vi "GetCurrentCharacter.vi"(8 "error in (no error)":errorcluster, 11 "TransformTokenizer in":refnum<class "TransformTokenizer.lvclass">) -> (0 "error out":errorcluster, 2 "Character":string, 3 "TransformTokenizer out":refnum<class "TransformTokenizer.lvclass">)   [LabVIEW 2019, in "TransformTokenizer.lvclass"]
uses:
  TransformTokenizer.lvclass
  TransformTokenizer.lvclass/TransformTokenizer.ctl
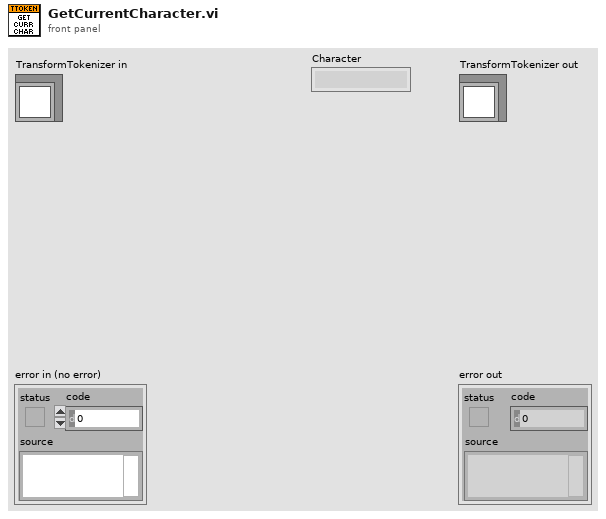
[diagram p1: front panel]
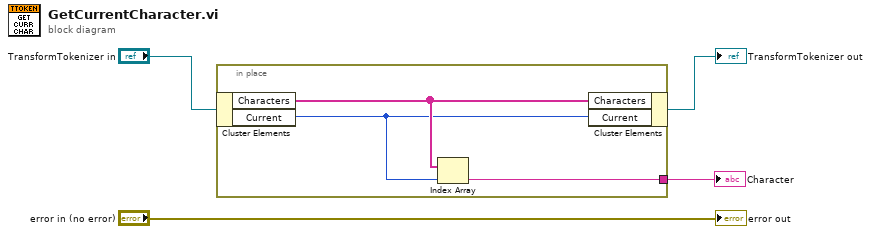
[diagram p0: block diagram]
diagram:
  n1 = in-place {
    in-place-border: [w5] -> w1
    n2 = in-place-cluster #1("TransformTokenizer in") -> ("Characters"=w7:string[], "Current"=w6:i32)
    n3 = Index Array(array=w7, index=w6) -> (element=w5:string)
    n4 = in-place-cluster #1("Characters"=w7, "Current"=w6) -> (→"TransformTokenizer out":refnum<class "TransformTokenizer.lvclass">)
  }
  "Character" <- w1
  "error out" <- "error in (no error)"
